vi "CLSUIP_CopyVIProjectItemHierarchy.vi"(8 "error in":errorcluster, 9 "Parent Types":string[](array[string]), 10 "Parent Names":string[](array[string]), 11 "StartingProjectItem":refnum<vi>) -> (0 "error out":errorcluster, 3 "NewParentItem":refnum<vi>)   [LabVIEW 2021]
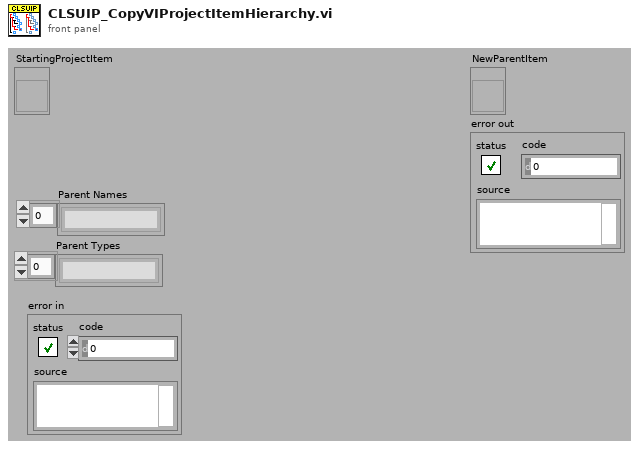
[diagram p1: front panel]
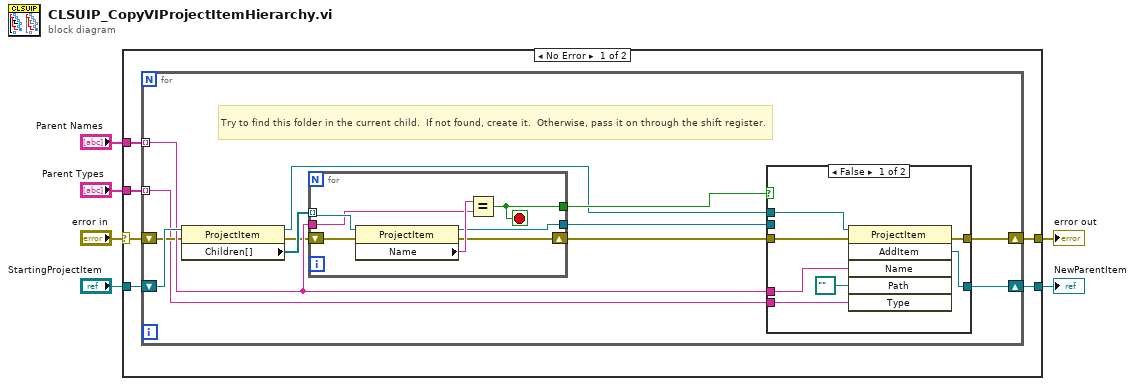
[diagram p0: block diagram]
diagram:
  n1 = case shown="No Error" "error in" {
    selector: "error in" -> [w7 w42]
    tunnel: "StartingProjectItem" -> [w12 w41]
    tunnel: "Parent Names" -> [w11 _]
    tunnel: "Parent Types" -> [w10 _]
    tunnel: [w9 w41] -> w3
    tunnel: [w8 w42] -> w2
    frame No Error {
      n2 = for {
        tunnel: w11 -> [w19] mode=indexing
        shift-right: [w20] -> w9
        shift-left: w12 -> [w24]
        shift-right: [w16] -> w8
        shift-left: w7 -> [w15]
        tunnel: w10 -> [w14] mode=indexing
        # "Try to find this folder in the current child.  If not found, create it.  Otherwise, pass it on through the shift register."
        n3 = property class="ProjectItem"(reference=w24, error in=w15) -> (reference out=w13:refnum<vi>, error out=w17:errorcluster, "Children[]"=w23:refnum<vi>[])
        n4 = for {
          tunnel: w23 -> [w40] mode=indexing
          tunnel: w19 -> [w38]
          tunnel: [w37] -> w22
          tunnel: [w36] -> w21
          shift-right: [w35] -> w18
          shift-left: w17 -> [w34]
          stop <- w37 stop-if-true
          n5 = property class="ProjectItem"(reference=w40, error in=w34) -> (reference out=w36:refnum<vi>, error out=w35:errorcluster, "Name"=w39:string)
          n6 = Equal?(x=w39, y=w38) -> (x = y?=w37:bool)
        }
        n7 = case shown="False" w22 {
          tunnel: w21 -> [_ w33]
          tunnel: [w29 w33] -> w20
          tunnel: w19 -> [w30 _]
          tunnel: w18 -> [w28 w32]
          tunnel: [w27 w32] -> w16
          tunnel: w14 -> [w26 _]
          tunnel: w13 -> [w25 _]
          frame False {
            n8 = invoke class="ProjectItem" method="AddItem"(reference=w25, error in=w28, "Name"=w30, "Path"=path "", "Type"=w26) -> (error out=w27:errorcluster, "AddItem"=w29:refnum<vi>)  [unwired: 1 in, 4 out]
          }
          frame True {
          }
        }
      }
    }
    frame Error {
    }
  }
  "NewParentItem" <- w3
  "error out" <- w2
